vi "Set Live Voltage.vi"(8 "error in":errorcluster, 10 "V":sgl, 11 "TEC 1090 in":refnum<class "Meerstetter TEC.lvclass">) -> (0 "error out":errorcluster, 3 "TEC 1090 out":refnum<class "Meerstetter TEC.lvclass">)   [LabVIEW 2014, in "Meerstetter Lib.lvlib" / "Meerstetter TEC.lvclass"]
uses:
  Meerstetter TEC.lvclass
  reusable/Session APIs/Serial/Serial Session.lvclass
  Configurable Device/Configurable Device.lvclass/Configurable Device.ctl
  Meerstetter TEC.lvclass/Meerstetter TEC.ctl
  Configurable Device/Read Log Session.vi
  Accessors/Read SerialSession.vi
  Configurable Device/Read ID.vi
  reusable/Session APIs/Serial/Public/Asynchronous Write.vi
  reusable/Session APIs/Serial/Public/Asynchronous Read.vi
  <userlib>/_Session Fwk/Session - Root.lvclass
  reusable/Session APIs/Session Log/System Log.lvclass
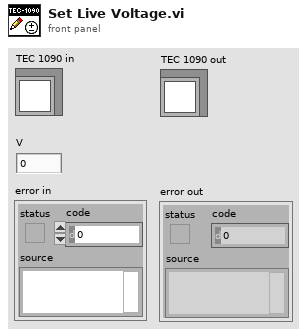
[diagram p1: front panel]
types:
  T1 = typedef "Session - Root.lvclass/Session Handle.ctl" = refnum<data-value>
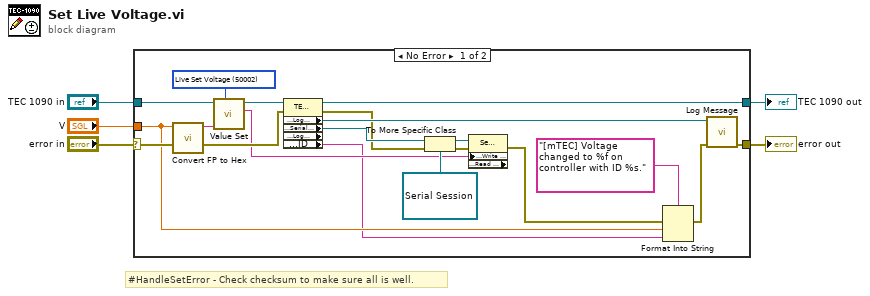
[diagram p0: block diagram]
diagram:
  # "#HandleSetError - Check checksum to make sure all is well."
  n1 = case shown="No Error" "error in" {
    selector: "error in" -> [w20 w26]
    tunnel: [w9 w26] -> w4
    tunnel: [w16 w25] -> w2
    tunnel: "TEC 1090 in" -> [w24 w25]
    tunnel: "V" -> [w14 _]
    frame No Error {
      w22 = u16 50002 items=["Input Selection"=2000, "Status"=2010, "Set Current"=2020, "Set Voltage"=2021, "Current Limitation"=2030, "Voltage Limitation"=2031, "Current Error Threshold"=2032, "Voltage Error Threshold"=2033, "Channel Baud Rate"=2050, "Response Delay"=2052, "Timeout"=2060, "Target Object Temperature"=3000, "Coarse Temp Ramp"=3003, "Proximity Width"=3002, "Kp"=3010, "Ti"=3011, "Td"=3012, "D Part Damping D1"=3013, "Live Enable"=50000, "Live Set Current"=50001, "Live Set Voltage"=50002, "Object Target Temperature"=50012, "Save Data to Flash"=108] ("Value Set")
      n2 = call "Convert FP to Hex.vi"("Number"=w14) -> ("hex integer string"=w23:string)  [unwired: 10 in]
      n3 = call "Value Set.vi"("Value Set"=w22, "Value"=w23, "TEC 1090"=w24) -> ("hex integer string"=w15:string, "TEC 1091"=w21:refnum<class "Meerstetter TEC.lvclass">)  [unwired: 7 in]
      n4 = property class="TEC 1090" props=["Accessors:Log Session", "Accessors:SerialSession", "Accessors:Log Session", "Accessors:ID"](reference=w21, error in=w20) -> (reference out=w16:refnum<class "Meerstetter TEC.lvclass">, error out=w6:errorcluster, "Accessors:Log Session"=w7:T1, "Accessors:SerialSession"=w8:T1, "Accessors:ID"=w10:string)  [unwired: 1 out]
      n5 = To More Specific Class(target class=refnum<data-value> refnum, reference=w8, error in=w6) -> (specific class reference=w18:refnum<data-value>, error out=w17:errorcluster)
      n6 = property class="Serial Session" props=["Public:Write - Asynchronous", "Public:Read - Asynchronous"](reference=w18, error in=w17, "Public:Write - Asynchronous"=w15) -> (error out=w12:errorcluster)  [unwired: 2 out]
      n7 = Format Into String(format string="[mTEC] Voltage changed to %f on controller with ID %s.", error in=w12, w14, w10) -> (error out=w13:errorcluster)  [unwired: 1 in, 1 out]
      n8 = call "Log Message.vi"("error in"=w13, "session in"=w7) -> ("error out"=w9:errorcluster)  [unwired: 8 in, 1 out]
    }
    frame Error {
    }
  }
  "error out" <- w4
  "TEC 1090 out" <- w2
